vi "Plot_Individual.vi"() -> ()   [LabVIEW 2019]
uses:
  <vilib>/Utility/file.llb/Read Delimited Spreadsheet (string).vi
panel:
  in  "Listbox":i32(listbox)
  out "Spectrum Data":cluster{dbl[], dbl[]}(graph) caption="XY Graph - Dark"
  out "Plotting":string
  in  "stop":bool
  in  "File Path":path
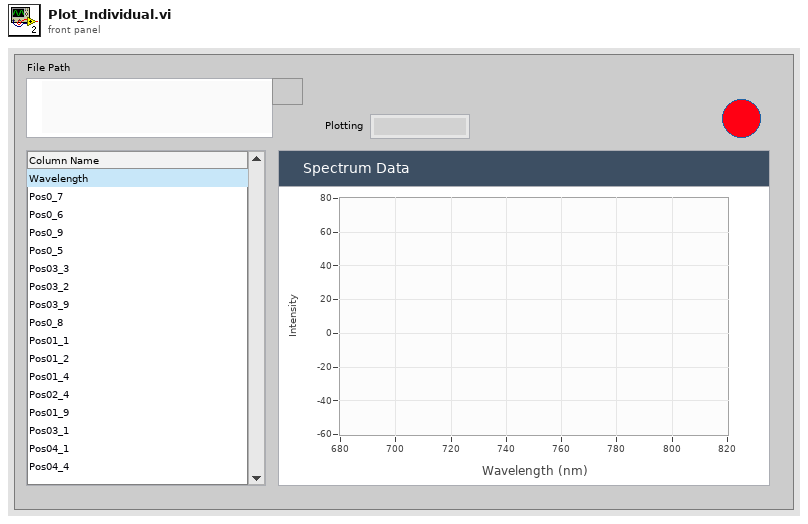
[diagram p1: front panel]
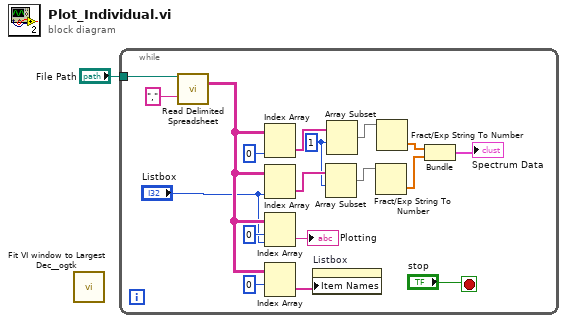
[diagram p0: block diagram]
diagram:
  n1 = call <userlib>:"Fit VI window to Largest Dec__ogtk.vi"() -> ()  [unwired: 6 in, 2 out]
  n2 = while {
    tunnel: "File Path" -> [w2]
    stop <- "stop" stop-if-true
    w12 = 1 ("index")
    n3 = call-poly <vilib>:"Read Delimited Spreadsheet.vi"("file path (dialog if empty)"=w2, "delimiter (\\t)"="," ("delimiter (\\t)")) -> ("all rows"=w6:string[][])  [unwired: 8 in, 5 out]
    n4 = Index Array(array=w6, index (col)=0 ("disabled index (col)")) -> (element=w14:string[])  [unwired: 1 in]
    n5 = Index Array(array=w6, index (col)="Listbox") -> (element=w13:string[])  [unwired: 1 in]
    n6 = Index Array(array=w6, index (row)=0 ("disabled index (row)"), index (col)="Listbox") -> (element=→"Plotting":string)
    n7 = Index Array(array=w6, index (row)=0) -> (element=w4:string[])  [unwired: 1 in]
    n8 = property on="Listbox" class="LstBox (strict)"("Item Names"=w4) -> ()  [unwired: 2 in, 2 out]
    n9 = Array Subset(array=w13, index=w12) -> (w10:string[])  [unwired: 1 in]
    n10 = Array Subset(array=w14, index=w12) -> (w11:string[])  [unwired: 1 in]
    n11 = Fract/Exp String To Number(string=w10) -> (number=w8:dbl[])  [unwired: 3 in, 1 out]
    n12 = Fract/Exp String To Number(string=w11) -> (number=w9:dbl[])  [unwired: 3 in, 1 out]
    n13 = Bundle(w9, w8) -> (→"Spectrum Data":cluster{dbl[], dbl[]})  [unwired: 1 in]
  }
